vi "main.vi"() -> ()   [LabVIEW 2010]
uses:
  <vilib>/Instr/_visa.llb/VISA Configure Serial Port (Instr).vi
panel:
  in  "数值调整":bool
  out "3轴平方和":dbl
  out "Z轴负值检测":bool
  out "?":cluster{"瞬时角速率":dbl, "瞬时角速率":dbl, "瞬时角速率":dbl}(graph)
  out "80":u8
  out "80":u8
  in  "?":bool
  in  "串口选择：":refnum<visa-resource-name>
  # "理论为128"
  # "理论为128"
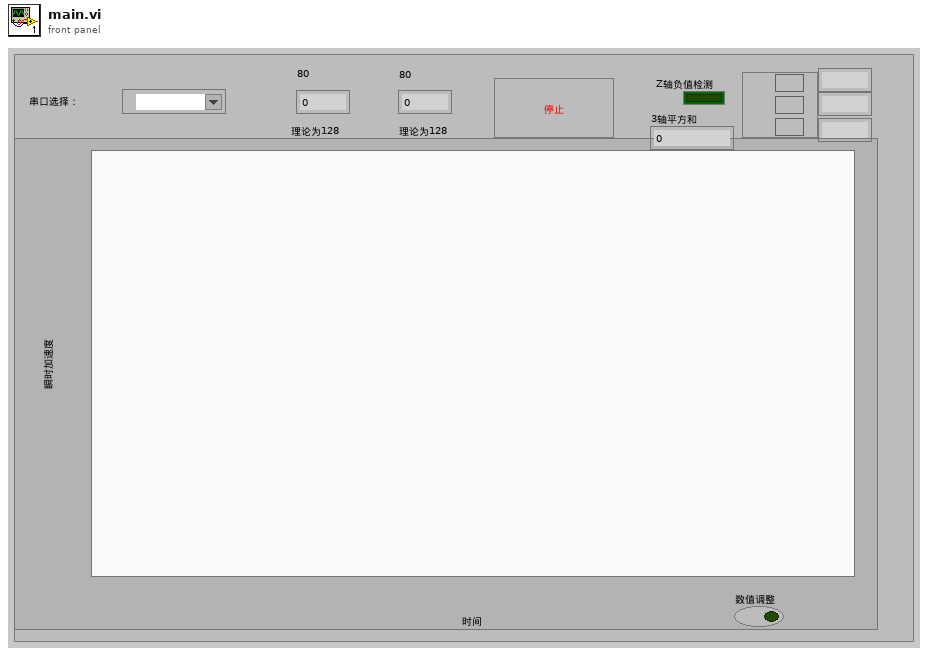
[diagram p1: front panel]
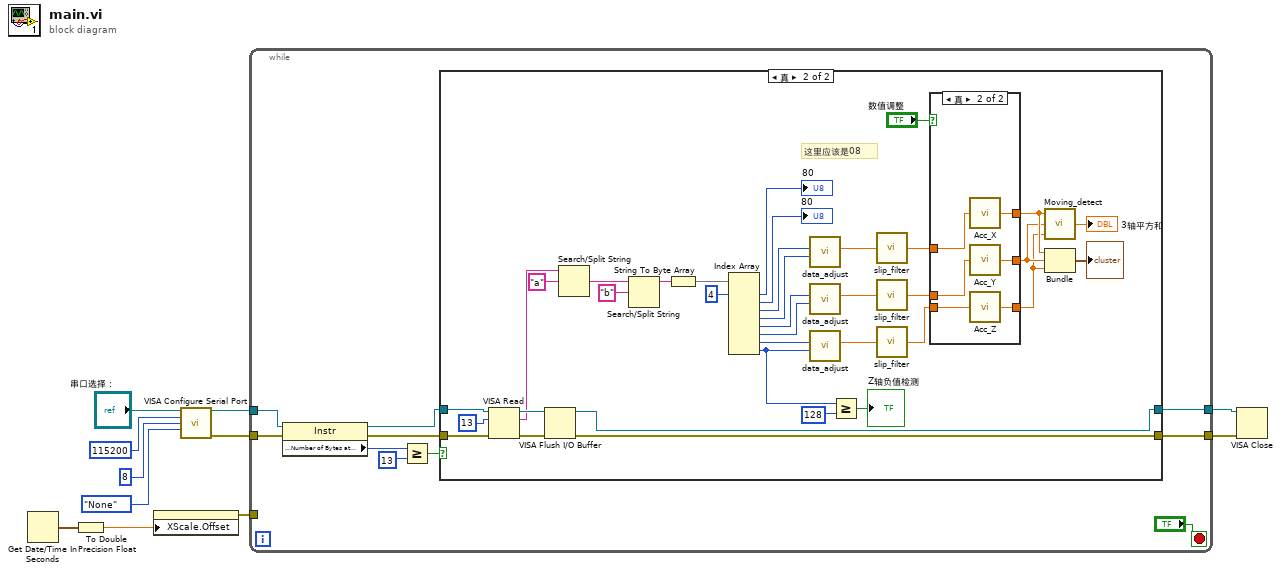
[diagram p0: block diagram]
diagram:
  n1 = Get Date/Time In Seconds() -> (seconds since 1Jan1904=w3:timestamp)
  n2 = To Double Precision Float(number=w3) -> (double precision float=w2:dbl)
  n3 = property class="WFChart (严格)"("XScale.Offset"=w2) -> (error out=w1:errorcluster)  [unwired: 2 in, 1 out]
  n4 = call-poly "VISA Configure Serial Port"("VISA resource name"="串口选择：", "baud rate (9600)"=u32 115200, "data bits (8)"=u16 8, "parity (0:none)"=enum16{"None", "Odd", "Even", "Mark", "Space"}."None") -> ("VISA resource name out"=w7:refnum<visa-resource-name>, "error out"=w6:errorcluster)  [unwired: 2 in, 8 out]
  n5 = while {
    tunnel: w7 -> [w21]
    tunnel: w6 -> [w20]
    tunnel: [w18] -> w5
    tunnel: [w17] -> w4
    tunnel: w1 -> [_]
    stop <- "?" stop-if-true
    n6 = property class="Instr"(reference=w21, error in=w20) -> (reference out=w14:refnum<visa-resource-name>, error out=w12:errorcluster, "Serial Settings:Number of Bytes at Serial Port"=w13:u32)
    n7 = Greater Or Equal?(x=w13, y=u32 13) -> (x >= y?=w15:bool)
    n8 = case shown="真" w15 {
      tunnel: w14 -> [w23 w59]
      tunnel: w12 -> [w22 w58]
      tunnel: [w23 w54] -> w18
      tunnel: [w22 w53] -> w17
      frame False {
      }
      frame True {
        # "这里应该是08"
        n9 = VISA Read(VISA resource name=w59, byte count=u32 13 ("字节总数"), error in (no error)=w58) -> (VISA resource name out=w56:refnum<visa-resource-name>, read buffer=w50:string, error out=w55:errorcluster)  [unwired: 1 out]
        n10 = VISA Flush I/O Buffer(VISA resource name=w56, error in (no error)=w55) -> (VISA resource name out=w54:refnum<visa-resource-name>, error out=w53:errorcluster)  [unwired: 1 out]
        n11 = Search/Split String(string=w50, search string/char (-)="a" ("搜索字符串/字符(-)")) -> (match + rest of string=w48:string)  [unwired: 1 in, 2 out]
        n12 = Search/Split String(string=w48, search string/char (-)="b" ("搜索字符串/字符(-)")) -> (substring before match=w46:string)  [unwired: 1 in, 2 out]
        n13 = String To Byte Array(string=w46) -> (unsigned byte array=w52:u8[])
        n14 = Index Array(array=w52, index #1=4 ("索引")) -> (element #1=→"80":u8, element #2=→"80":u8, element #3=w40:u8, element #4=w39:u8, element #5=w43:u8, element #6=w37:u8, element #7=w38:u8, element #8=w36:u8)  [unwired: 7 in]
        n15 = call "data_adjust.vi"("数据高位"=w39, "数据低位"=w40) -> ("瞬时加速度值"=w34:dbl)  [unwired: 9 in]
        n16 = call "data_adjust.vi"("数据高位"=w37, "数据低位"=w43) -> ("瞬时加速度值"=w33:dbl)  [unwired: 9 in]
        n17 = call "data_adjust.vi"("数据高位"=w36, "数据低位"=w38) -> ("瞬时加速度值"=w35:dbl)  [unwired: 9 in]
        n18 = Greater Or Equal?(x=w36, y=u8 128 ("元素")) -> (x >= y?=→"Z轴负值检测":bool)
        n19 = call "slip_filter.vi"("平滑滤波输入值"=w34) -> ("平滑滤波输出值"=w30:dbl)
        n20 = call "slip_filter.vi"("平滑滤波输入值"=w33) -> ("平滑滤波输出值"=w29:dbl)
        n21 = call "slip_filter.vi"("平滑滤波输入值"=w35) -> ("平滑滤波输出值"=w28:dbl)
        n22 = case shown="真" "数值调整" {
          tunnel: w30 -> [w62 w68]
          tunnel: [w62 w67] -> w27
          tunnel: w29 -> [w61 w66]
          tunnel: [w61 w65] -> w26
          tunnel: w28 -> [w60 w64]
          tunnel: [w60 w63] -> w25
          frame False {
          }
          frame True {
            n23 = call "Acc_X.vi"("x_ini"=w68) -> ("x_Acc"=w67:dbl)
            n24 = call "Acc_Y.vi"("y_ini"=w66) -> ("y_Acc"=w65:dbl)
            n25 = call "Acc_Z.vi"("z_ini"=w64) -> ("z_Acc"=w63:dbl)
          }
        }
        n26 = call "Moving_detect.vi"("Z"=w25, "Y"=w26, "X"=w27) -> ("3轴平方和"=→"3轴平方和":dbl)
        n27 = Bundle("x_Acc"=w27, "y_Acc"=w26, "z_Acc"=w25) -> (→"?":cluster{"x_Acc":dbl, "y_Acc":dbl, "z_Acc":dbl})  [unwired: 1 in]
      }
    }
  }
  n28 = VISA Close(VISA resource name=w5, error in (no error)=w4) -> ()  [unwired: 1 out]
